vi "merFISH_set_pressure_to_zero.vi"(2 "error in":errorcluster, 3 "queue pump":refnum<queue>) -> (0 "error out":errorcluster)   [LabVIEW 2015]
uses:
  CONTROLS/Q_PUMP_element.ctl
  GLOBAL/Global_ABORT.vi
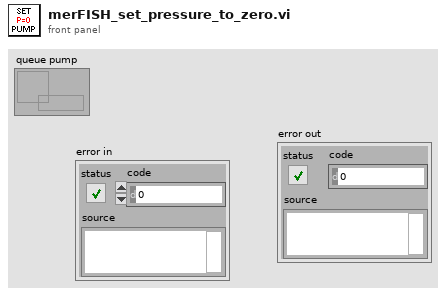
[diagram p1: front panel]
types:
  T1 = typedef "Q_PUMP_element.ctl" = cluster{"variant":variant, "Instruction":enum16{"PUMP_idle", "PUMP_initialize", "PUMP_error", "PUMP_security_stop", "PUMP_read_pressure", "PUMP_change_pressure", "PUMP_init_merFISH", "PUMP_change_presure_merFISH", "PUMP_zero_pressure_merFISH", "PUMP_close_merFISH", "PUMP_stop"}}
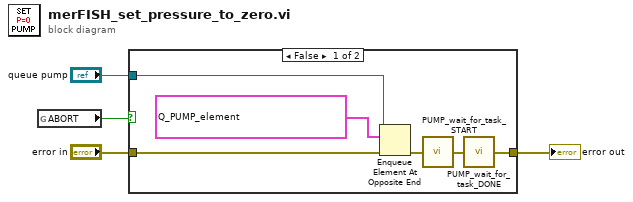
[diagram p0: block diagram]
diagram:
  n1 = global read "Global_ABORT.vi" "ABORT"() -> (w2:bool)
  n2 = case shown="False" w2 {
    tunnel: [w10 w11] -> w4
    tunnel: "queue pump" -> [w9 _]
    tunnel: "error in" -> [w6 w11]
    frame False {
      n3 = Enqueue Element At Opposite End(queue=w9, element=T1 {"variant"=variant, "Instruction"=enum."PUMP_zero_pressure_merFISH"}, error in (no error)=w6) -> (error out=w8:errorcluster)  [unwired: 1 in, 2 out]
      n4 = call "PUMP_wait_for_task_START.vi"("error in"=w8) -> ("error out"=w7:errorcluster)
      n5 = call "PUMP_wait_for_task_DONE.vi"("error in"=w7) -> ("error out"=w10:errorcluster)
    }
    frame True {
    }
  }
  "error out" <- w4
